vi "alertdisp.vi"() -> ()   [LabVIEW 2015]
uses:
  veloster/G_rio.vi
panel:
  out "Control":bool
  out "Gas/Brake":bool
  out "Steering":bool
  out "Laser":bool
  out "GPS":bool
  out "CAN":bool
  out "Camera":bool
  out "E - STOP":bool
  out "Auto":bool
  out "Run":bool
  out "Count Control":i32
  out "Count Laser":i32
  out "Count GPS":i32
  out "Count CAN":i32
  out "Count camera":i32
  # "KAIST EURECAR"
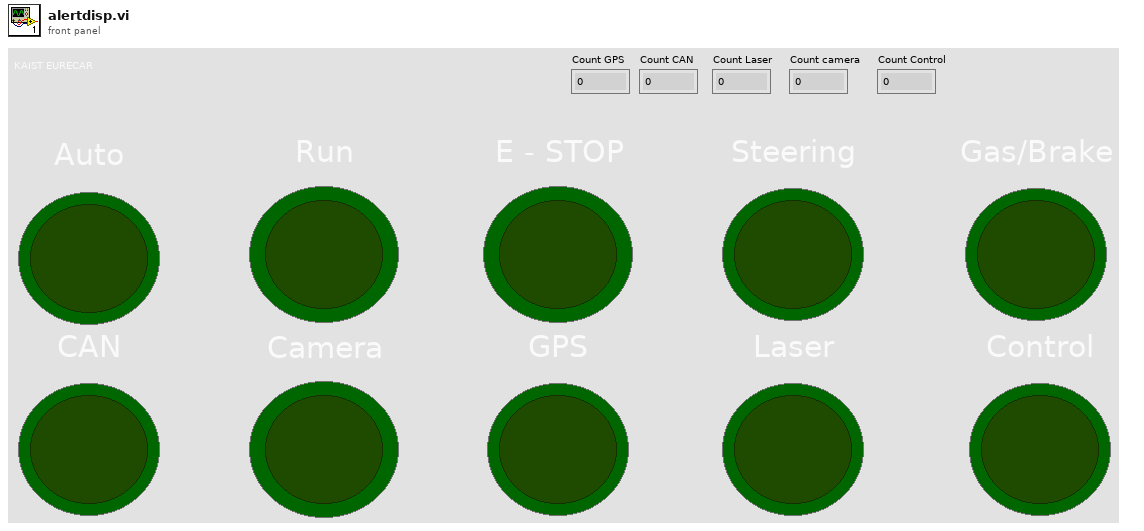
[diagram p1: front panel]
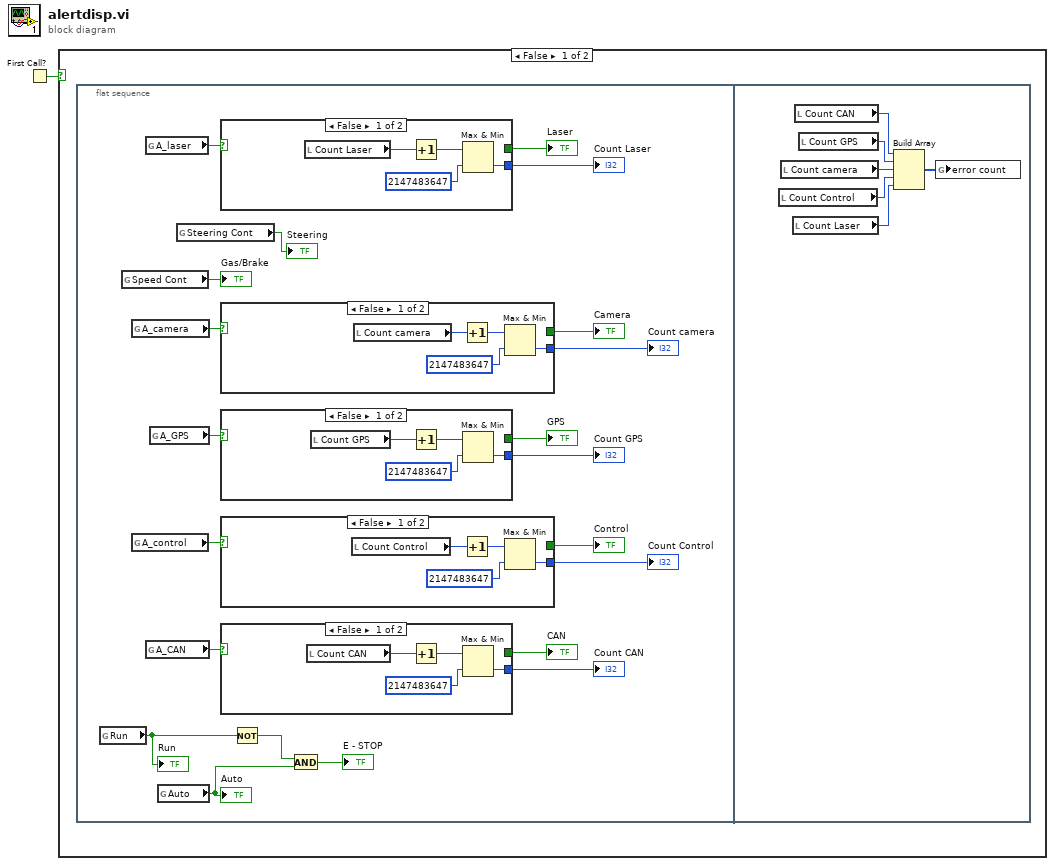
[diagram p0: block diagram]
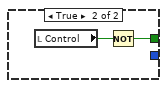
[diagram p2: hidden frame]
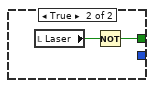
[diagram p3: hidden frame]
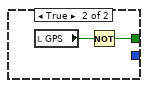
[diagram p4: hidden frame]
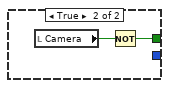
[diagram p5: hidden frame]
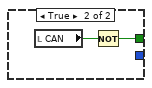
[diagram p6: hidden frame]
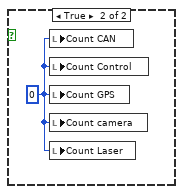
[diagram p7: hidden frame]
diagram:
  n1 = First Call?() -> (First Call?: T/F=w1:bool)
  n2 = case shown="False" w1 {
    frame False {
      n3 = flat-sequence {
        frame #0 {
          n4 = global read "G_rio.vi" "Run"() -> (w22:bool)
          "Run" <- w22
          n5 = global read "G_rio.vi" "Speed Cont"() -> (→"Gas/Brake":bool)
          n6 = global read "G_rio.vi" "A_camera"() -> (w16:bool)
          n7 = global read "G_rio.vi" "A_control"() -> (w2:bool)
          n8 = global read "G_rio.vi" "A_laser"() -> (w12:bool)
          n9 = global read "G_rio.vi" "A_CAN"() -> (w18:bool)
          n10 = global read "G_rio.vi" "A_GPS"() -> (w14:bool)
          n11 = global read "G_rio.vi" "Auto"() -> (w20:bool)
          "Auto" <- w20
          n12 = global read "G_rio.vi" "Steering Cont"() -> (→"Steering":bool)
          n13 = case shown="False" w12 {
            tunnel: [_ w33] -> w11
            tunnel: [w29 _] -> w6
            frame False {
              n14 = local read "Count Laser"() -> (w32:i32)
              n15 = Increment(x=w32) -> (x+1=w31:i32)
              n16 = Max & Min(x=w31, y=2147483647) -> (min(x,y)=w29:i32)  [unwired: 1 out]
            }
            frame True {
              n17 = local read "Laser"() -> (w34:bool)
              n18 = Not(x=w34) -> (.not. x?=w33:bool)
            }
          }
          "Laser" <- w11
          "Count Laser" <- w6
          n19 = case shown="False" w16 {
            tunnel: [_ w45] -> w15
            tunnel: [w41 _] -> w8
            frame False {
              n20 = local read "Count camera"() -> (w44:i32)
              n21 = Increment(x=w44) -> (x+1=w42:i32)
              n22 = Max & Min(x=w42, y=2147483647) -> (min(x,y)=w41:i32)  [unwired: 1 out]
            }
            frame True {
              n23 = local read "Camera"() -> (w46:bool)
              n24 = Not(x=w46) -> (.not. x?=w45:bool)
            }
          }
          "Camera" <- w15
          "Count camera" <- w8
          n25 = case shown="False" w14 {
            tunnel: [_ w39] -> w13
            tunnel: [w35 _] -> w5
            frame False {
              n26 = local read "Count GPS"() -> (w38:i32)
              n27 = Increment(x=w38) -> (x+1=w37:i32)
              n28 = Max & Min(x=w37, y=2147483647) -> (min(x,y)=w35:i32)  [unwired: 1 out]
            }
            frame True {
              n29 = local read "GPS"() -> (w40:bool)
              n30 = Not(x=w40) -> (.not. x?=w39:bool)
            }
          }
          "GPS" <- w13
          "Count GPS" <- w5
          n31 = case shown="False" w2 {
            tunnel: [_ w27] -> w3
            tunnel: [w23 _] -> w4
            frame False {
              n32 = local read "Count Control"() -> (w26:i32)
              n33 = Increment(x=w26) -> (x+1=w24:i32)
              n34 = Max & Min(x=w24, y=2147483647) -> (min(x,y)=w23:i32)  [unwired: 1 out]
            }
            frame True {
              n35 = local read "Control"() -> (w28:bool)
              n36 = Not(x=w28) -> (.not. x?=w27:bool)
            }
          }
          "Control" <- w3
          "Count Control" <- w4
          n37 = case shown="False" w18 {
            tunnel: [_ w51] -> w17
            tunnel: [w48 _] -> w7
            frame False {
              n38 = local read "Count CAN"() -> (w50:i32)
              n39 = Increment(x=w50) -> (x+1=w49:i32)
              n40 = Max & Min(x=w49, y=2147483647) -> (min(x,y)=w48:i32)  [unwired: 1 out]
            }
            frame True {
              n41 = local read "CAN"() -> (w52:bool)
              n42 = Not(x=w52) -> (.not. x?=w51:bool)
            }
          }
          "CAN" <- w17
          "Count CAN" <- w7
          n43 = Not(x=w22) -> (.not. x?=w21:bool)
          n44 = And(x=w21, y=w20) -> (x .and. y?=→"E - STOP":bool)
        }
        frame #1 {
          n45 = local read "Count Control"() -> (w55:i32)
          n46 = local read "Count camera"() -> (w56:i32)
          n47 = local read "Count Laser"() -> (w54:i32)
          n48 = local read "Count CAN"() -> (w58:i32)
          n49 = local read "Count GPS"() -> (w57:i32)
          n50 = Build Array(w58, w57, w56, w55, w54) -> (w53:i32[])
          n51 = global write "G_rio.vi" "error count"(w53) -> ()
        }
      }
    }
    frame True {
      w59 = 0 ("Count GPS")
      n52 = local write "Count CAN"(w59) -> ()
      n53 = local write "Count Control"(w59) -> ()
      n54 = local write "Count GPS"(w59) -> ()
      n55 = local write "Count camera"(w59) -> ()
      n56 = local write "Count Laser"(w59) -> ()
    }
  }
